vi "Store Static VI References for Subpanel.vi"(8 "error in (no error)":errorcluster, 11 "VacuumLine Configuration in":refnum<class "VacuumLine Configuration.lvclass">) -> (0 "error out":errorcluster, 3 "VacuumLine Configuration out":refnum<class "VacuumLine Configuration.lvclass">)   [LabVIEW 2016, in "Hardware.lvlib" / "VacuumLine.lvlib" / "VacuumLine Configuration.lvclass"]
uses:
  <userlib>/Common Components/Hardware/Abstract System/VacuumLine/VacuumLine Config/VacuumLine Configuration.lvclass
  <userlib>/Configuration Dialog Actor/Configuration.lvclass
  <userlib>/Common Components/Hardware/Motor/Motor Config/Motor Configuration.lvclass
  C:/Program Files (x86)/National Instruments/LabVIEW 2016/user.lib/Configuration Dialog Actor/Configuration.lvclass
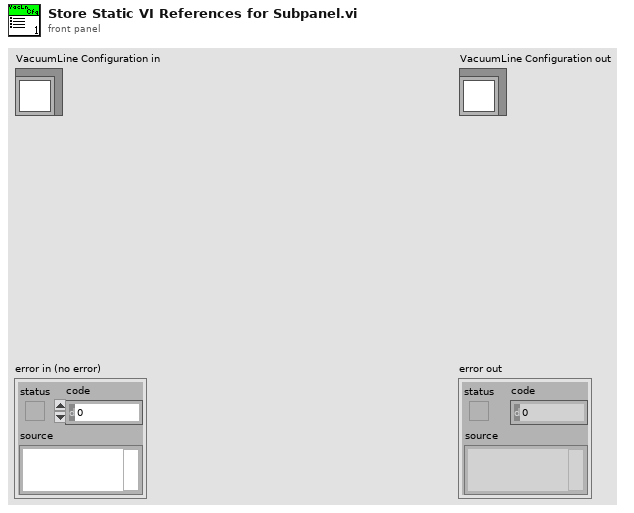
[diagram p1: front panel]
types:
  T1 = typedef "Configuration.lvlib/Configuration.lvclass/Data Retrieved by Lookup Table.ctl" = cluster{"VI Refnum":refnum<vi>, "Help Text":string}
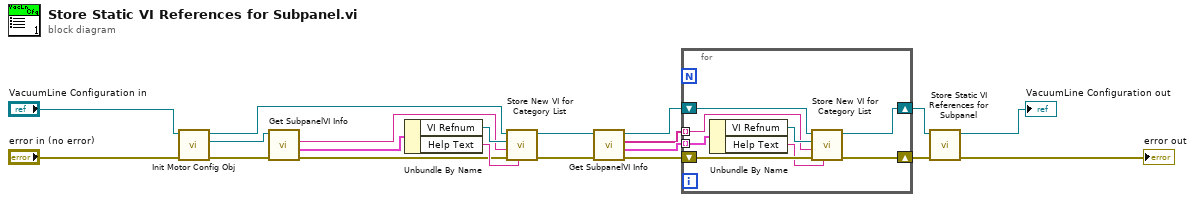
[diagram p0: block diagram]
diagram:
  n1 = call <userlib>:"Init Motor Config Obj.vi"("error in (no error)"="error in (no error)", "VacuumLine Configuration in"="VacuumLine Configuration in") -> ("error out"=w4:errorcluster, "Motor Config Obj"=w1:refnum<class "Motor Configuration.lvclass">, "VacuumLine Configuration out"=w3:refnum<class "VacuumLine Configuration.lvclass">)  [unwired: 7 in]
  n2 = call-dynamic "Get SubpanelVI Info.vi"("error in (no error)"=w4, "Motor Configuration in"=w1) -> ("error out"=w5:errorcluster, "Subpanel VI data"=w18:T1, "Category string"=w14:string)  [unwired: 6 in, 1 out]
  n3 = Unbundle By Name(w18) -> ("VI Refnum"=w16:refnum<vi>, "Help Text"=w15:string)
  n4 = call <userlib>:"Store New VI for Category List.vi"("Help Text"=w15, "error in (no error)"=w5, "String"=w14, "VI Refnum"=w16, "Configuration in"=w3) -> ("error out"=w8:errorcluster, "Configuration out"=w17:refnum<class "VacuumLine Configuration.lvclass">)  [unwired: 5 in]
  n5 = call-dynamic "Get SubpanelVI Info.vi"("error in (no error)"=w8, "VacuumLine Configuration in"=w17) -> ("error out"=w7:errorcluster, "Array of Subpanel VI data"=w13:T1[], "Array of Category string"=w12:string[], "VacuumLine Configuration out"=w11:refnum<class "VacuumLine Configuration.lvclass">)  [unwired: 6 in]
  n6 = for {
    tunnel: w13 -> [w24] mode=indexing
    tunnel: w12 -> [w21] mode=indexing
    shift-right: [w27] -> w9
    shift-left: w7 -> [w28]
    shift-right: [w25] -> w10
    shift-left: w11 -> [w26]
    n7 = Unbundle By Name(w24) -> ("VI Refnum"=w23:refnum<vi>, "Help Text"=w22:string)
    n8 = call <userlib>:"Store New VI for Category List.vi"("Help Text"=w22, "error in (no error)"=w28, "String"=w21, "VI Refnum"=w23, "Configuration in"=w26) -> ("error out"=w27:errorcluster, "Configuration out"=w25:refnum<class "VacuumLine Configuration.lvclass">)  [unwired: 5 in]
  }
  n9 = call-parent "Store Static VI References for Subpanel.vi"("error in (no error)"=w9, "Configuration in"=w10) -> ("error out"=→"error out":errorcluster, "Configuration out"=→"VacuumLine Configuration out":refnum<class "VacuumLine Configuration.lvclass">)  [unwired: 8 in]
